vi "Do Request.vi"(7 "Arguments":refnum<class "Arguments.lvclass">, 8 "error in (no error)":errorcluster, 10 "Request In":refnum<class "Request.lvclass">, 11 "Test Index in":refnum<class "Test Index.lvclass">) -> (0 "error out":errorcluster, 1 "Response":refnum<class "Response.lvclass">, 2 "Request":refnum<class "Request.lvclass">)   [LabVIEW 2020, in "Test Index.lvclass"]
uses:
  Test Index.lvclass
  <vilib>/IlluminatedG/IG HTTP Utils/HTTP Utils/Request/Request.lvclass
  <vilib>/IlluminatedG/IG HTTP Utils/HTTP Utils/Response/Response.lvclass
  HTTP Server/Arguments/Arguments.lvclass
  c41d861c-1b9b-49d8-b440-13b65674a8cc.vi
  53043089-065a-48e9-b126-a7fdc944236f.vi
  HTTP Server/Arguments/Get Arg Map.vi
  <vilib>/Utility/error.llb/Error Cluster From Error Code.vi
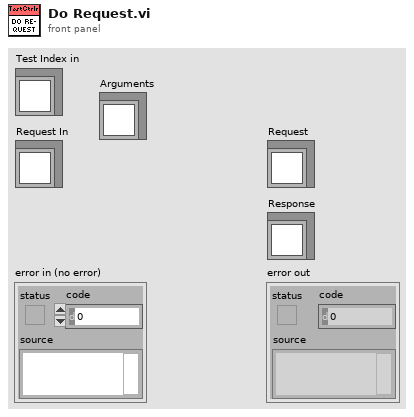
[diagram p1: front panel]
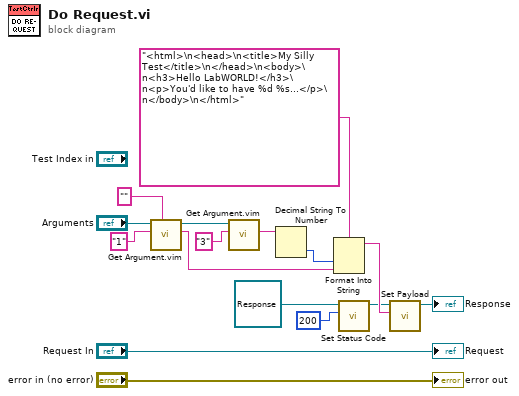
[diagram p0: block diagram]
diagram:
  n1 = call "Get Argument.vim"("Service / Type (String)"="" ("Name for Type (Service)"), "Name for Type (Service)"="1", "Arguments in"="Arguments") -> ("Value"=w7:string, "Arguments out"=w10:refnum<class "Arguments.lvclass">)  [unwired: 6 in, 1 out]
  n2 = call "Get Argument.vim"("Name for Type (Service)"="3", "Arguments in"=w10) -> ("Value"=w2:string)  [unwired: 7 in, 2 out]
  n3 = Decimal String To Number(string=w2) -> (number=w1:i32)  [unwired: 2 in, 1 out]
  n4 = Format Into String(format string="<html>\n<head>\n<title>My Silly Test</title>\n</head>\n<body>\n<h3>Hello LabWORLD!</h3>\n<p>You'd like to have %d %s...</p>\n</body>\n</html>", w1, w7) -> (resulting string=w13:string)  [unwired: 2 in, 1 out]
  n5 = call <vilib>:"Set Status Code.vi"("Status Code"=u16 200, "Response in"=refnum<class "Response.lvclass"> refnum) -> ("Response out"=w6:refnum<class "Response.lvclass">)  [unwired: 8 in, 1 out]
  n6 = call <vilib>:"Set Payload.vi"("Payload"=w13, "Response in"=w6) -> ("Response out"=→"Response":refnum<class "Response.lvclass">)  [unwired: 8 in, 1 out]
  "error out" <- "error in (no error)"
  "Request" <- "Request In"
